vi "MakeFileNameValid.vi"(8 "Fehler (Eingang, kein Fehler)":errorcluster, 11 "Dateiname:":string) -> (0 "Fehler (Ausgang)":errorcluster, 3 "result string":string)   [LabVIEW 2015, in "allgemeine Sub-VIs.lvlib"]
uses:
  allgemeine Sub-VIs.lvlib
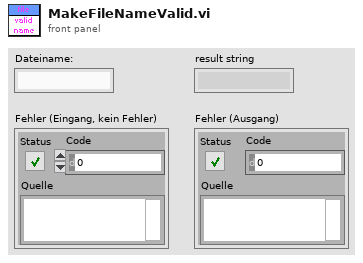
[diagram p1: front panel]
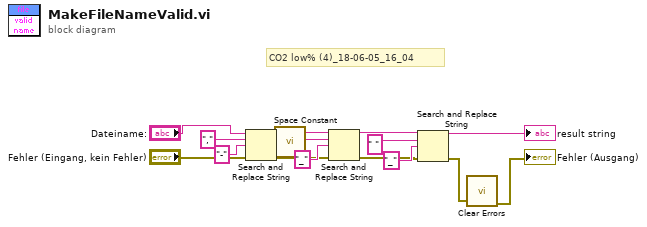
[diagram p0: block diagram]
diagram:
  # "CO2 low% (4)_18-06-05_16_04"
  n1 = Search and Replace String(input string="Dateiname:", search string="," ("Such-String"), replace string="-" ("Ersetzungs-String (\"\")"), error in="Fehler (Eingang, kein Fehler)") -> (result string=w8:string, error out=w10:errorcluster)  [unwired: 4 in, 2 out]
  n2 = call <vilib>:"Space Constant.vi"() -> ("String"=w4:string)
  n3 = Search and Replace String(input string=w8, search string=w4, replace string="_" ("Ersetzungs-String (\"\")"), error in=w10) -> (result string=w7:string, error out=w9:errorcluster)  [unwired: 4 in, 2 out]
  n4 = Search and Replace String(input string=w7, search string=" " ("Ersetzungs-String (\"\")"), replace string="_" ("Ersetzungs-String (\"\")"), error in=w9) -> (result string=→"result string":string, error out=w2:errorcluster)  [unwired: 4 in, 2 out]
  n5 = call <vilib>:"Clear Errors.vi"("error in (no error)"=w2) -> ("error out"=→"Fehler (Ausgang)":errorcluster)  [unwired: 5 in, 1 out]
